vi "Generacion_contorno.vi"() -> ()   [LabVIEW 2017]
uses:
  <vilib>/Motion/Express/_s/nimc.fb.straightLineMove.startStraightLineMove.axis.modeAbsolute.0.vi
  <vilib>/Motion/Express/_s/nimc.fb.read.readExecutionData.axis.vi
  <vilib>/Motion/Express/_s/nimc.fb.contourMove.startContourMove.axis.modeFinite.vi
  <vilib>/Motion/BlockNode/FB.NIMotion.xnode
  <vilib>/Motion/Express/_s/nimc.fb.contourMove.splineType.ctl
panel:
  in  "Stop Button":bool
  in  "Play Button":bool
  out "Eje x":dbl(slide) scale=-100.0..100.0
  out "Exje Y":dbl(slide)=-0.0 scale=-100.0..100.0
  out "XY Graph":cluster{dbl[], dbl[]}(graph)
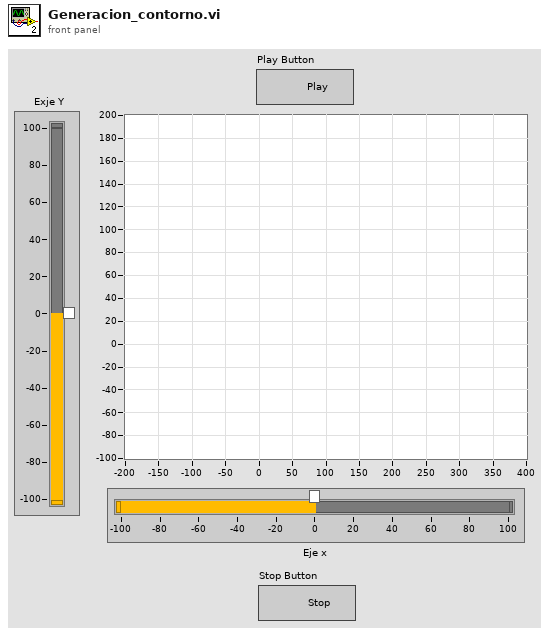
[diagram p1: front panel]
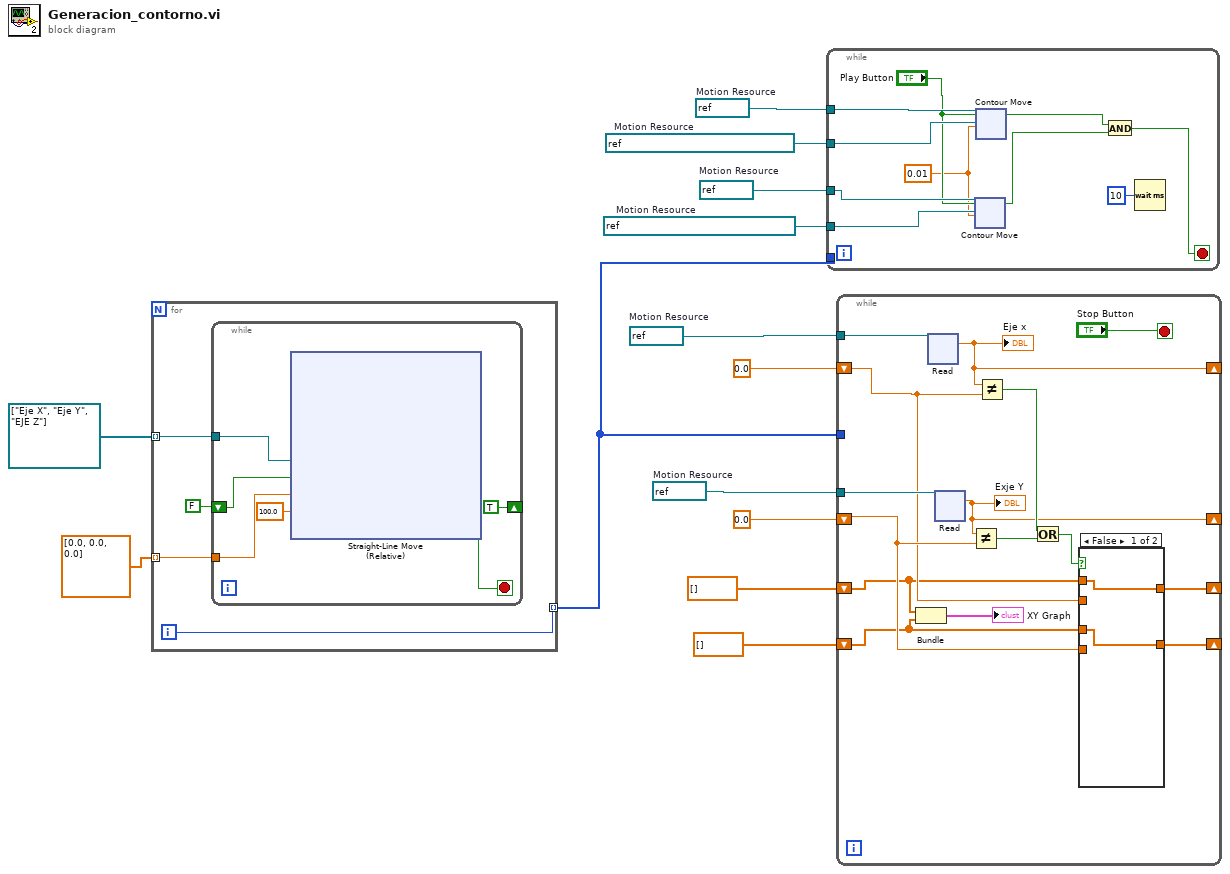
[diagram p0: block diagram]
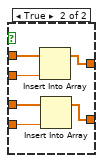
[diagram p2: hidden frame]
diagram:
  w2 = refnum<k21> "TablaX"  # Motion Resource
  w1 = refnum<k21> "TablaY"  # Motion Resource
  w3 = refnum<k21> "Eje Y"  # Motion Resource
  w5 = refnum<k21> "Eje X"  # Motion Resource
  w12 = refnum<k21> "Eje Y"  # Motion Resource
  w13 = refnum<k21> "Eje X"  # Motion Resource
  n1 = for {
    tunnel: refnum<k21>[] ["Eje X", "Eje Y", "EJE Z"] -> [w15] mode=indexing
    tunnel: dbl[] [0.0, 0.0, 0.0] -> [w16] mode=indexing
    tunnel: [w14] -> w4 mode=indexing
    i -> [w14]
    n2 = while {
      shift-right: [TRUE] -> _
      shift-left: FALSE -> [w23]
      tunnel: w16 -> [w20]
      tunnel: w15 -> [w19]
      stop <- w22 stop-if-true
      n3 = xnode "Straight-Line Move\n(Relative)"("resource"=w19, "execute"=w23, "position"=w20, "velocity"=100.0) -> ("done"=w22:bool)  [unwired: 2 in, 2 out]
    }
  }
  n4 = while {
    tunnel: w5 -> [w50]
    tunnel: w4 -> [_]
    tunnel: w3 -> [w47]
    tunnel: w2 -> [w46]
    tunnel: w1 -> [w45]
    stop <- w48 stop-if-true
    w42 = 0.01 ("interval")
    n5 = xnode "Contour Move"("resource"=w47, "execute"="Play Button", "table"=w45, "interval"=w42) -> ("done"=w44:bool)  [unwired: 2 in, 5 out]
    n6 = xnode "Contour Move"("resource"=w50, "execute"="Play Button", "table"=w46, "interval"=w42) -> ("done"=w49:bool)  [unwired: 2 in, 5 out]
    n7 = And(x=w49, y=w44) -> (x .and. y?=w48:bool)
    n8 = Wait (ms)(milliseconds to wait=u32 10) -> ()  [unwired: 1 out]
  }
  n9 = while {
    tunnel: w13 -> [w109]
    tunnel: w12 -> [w108]
    shift-right: [w97] -> _
    shift-left: 0.0 ("position") -> [w101]
    shift-right: [w96] -> _
    shift-left: 0.0 ("position") -> [w102]
    shift-right: [w104] -> _
    shift-left: dbl[] [] -> [w100]
    shift-right: [w103] -> _
    shift-left: dbl[] [] -> [w99]
    tunnel: w4 -> [_]
    stop <- "Stop Button" stop-if-true
    n10 = Bundle(w100, w99) -> (→"XY Graph":cluster{dbl[], dbl[]})  [unwired: 1 in]
    n11 = xnode "Read"("resource"=w109) -> ("position"=w97:dbl)  [unwired: 2 in, 7 out]
    "Eje x" <- w97
    n12 = xnode "Read"("resource"=w108) -> ("position"=w96:dbl)  [unwired: 2 in, 7 out]
    "Exje Y" <- w96
    n13 = Not Equal?(x=w96, y=w102) -> (x != y?=w106:bool)
    n14 = Not Equal?(x=w97, y=w101) -> (x != y?=w107:bool)
    n15 = Or(x=w107, y=w106) -> (x .or. y?=w105:bool)
    n16 = case shown="False" w105 {
      tunnel: w100 -> [w111 w117]
      tunnel: [w111 w116] -> w104
      tunnel: w99 -> [w110 w115]
      tunnel: [w110 w114] -> w103
      tunnel: w102 -> [_ w113]
      tunnel: w101 -> [_ w112]
      frame False {
      }
      frame True {
        n17 = Insert Into Array(array=w117, new element=w112) -> (w116:dbl[])  [unwired: 1 in]
        n18 = Insert Into Array(array=w115, new element=w113) -> (w114:dbl[])  [unwired: 1 in]
      }
    }
  }
